vi "InputPATH   OutputIMAGE.vi"(11 "appended path":path) -> (0 "error out":errorcluster, 3 "Refnum out":T1)   [LabVIEW 2011]
uses:
  <vilib>/vision/Image Controls.llb/IMAQ Image.ctl
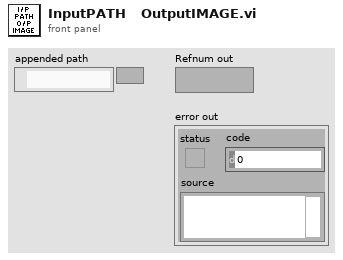
[diagram p1: front panel]
types:
  T1 = typedef "IMAQ Image.ctl" = refnum<image>
  T2 = enum32{"8 bits", "16 bits", "Float", "Complex", "RGB Chunky", "Compressed"}
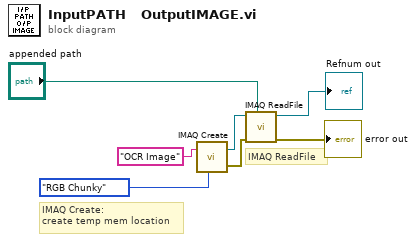
[diagram p0: block diagram]
diagram:
  # "IMAQ Create:\ncreate temp mem location"
  # "IMAQ ReadFile"
  n1 = call "IMAQ Create"("Image Name"="OCR Image", "Image Type"=T2."RGB Chunky") -> ("New Image"=w3:T1, "error out"=w5:errorcluster)  [unwired: 2 in, 1 out]
  n2 = call "IMAQ ReadFile"("File Path"="appended path", "error in (no error)"=w5, "Image"=w3) -> ("error out"=→"error out":errorcluster, "Image Out"=→"Refnum out":T1)  [unwired: 2 in, 5 out]
